vi "TPNT_file2fits.vi"(7 "mext":bool, 8 "error in (no error)":errorcluster, 9 "action":T1(ring)=enum."get all", 10 "number of Extensions":u16, 11 "filename":path=path "/home/bonati/panview_current/fpas/_decam45/config/TPNT_INFO.tpl") -> (0 "error out":errorcluster, 1 "flat keys":string[][](table), 2 "number of keywords":i32[](array[numeric]), 3 "Keywords":string[][][](array[string]), 5 "number of Extensions out":u16)   [LabVIEW 2016]
doc: "test"
panel:
  out "Extensions":i32[][](array[numeric])
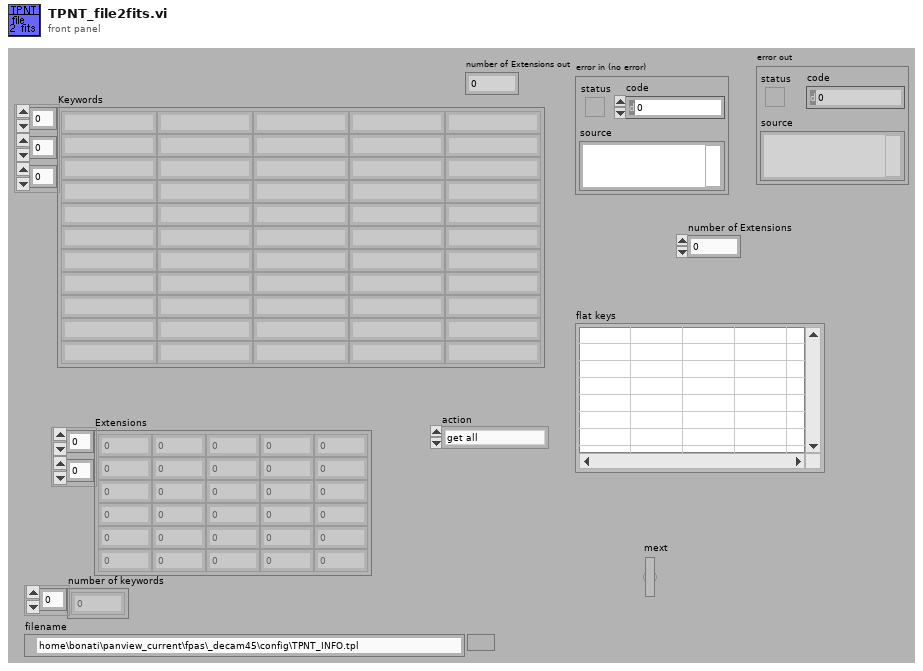
[diagram p1: front panel]
types:
  T1 = enum16{"read from file", "get all", "clear all", "set file"}
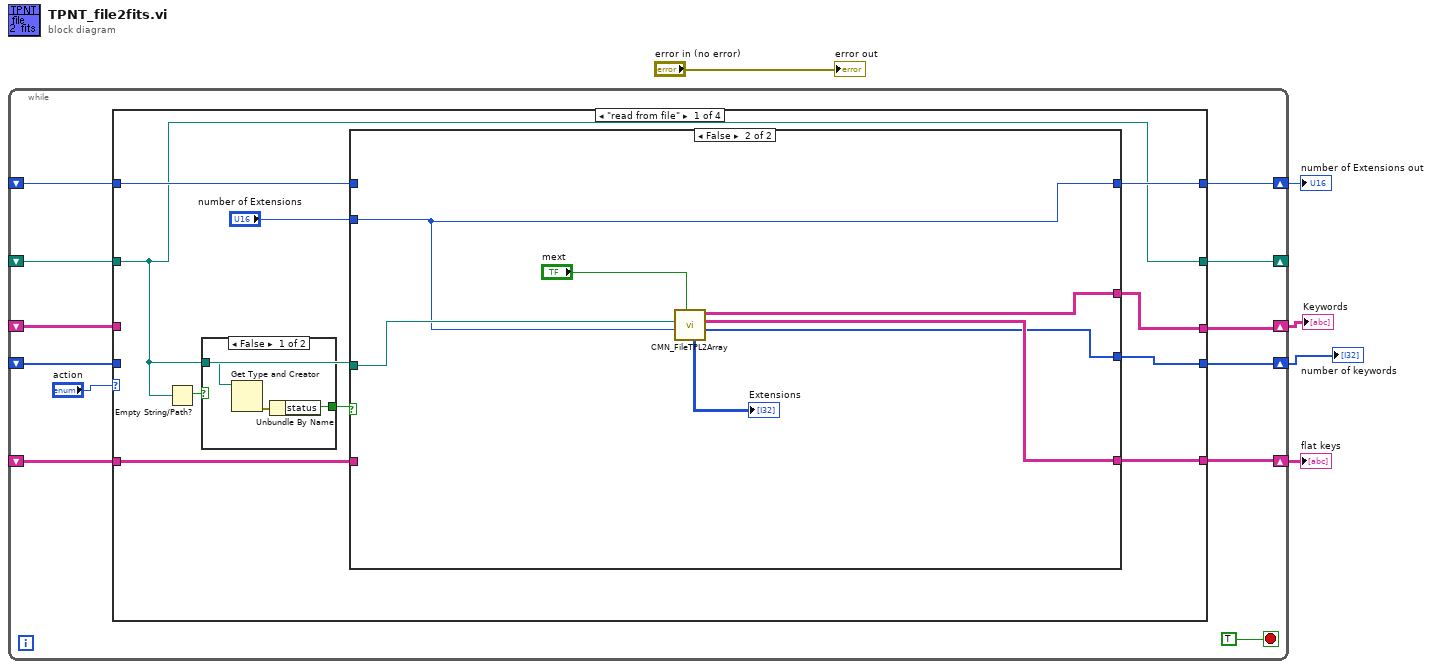
[diagram p0: block diagram]
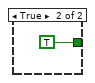
[diagram p2: hidden frame]
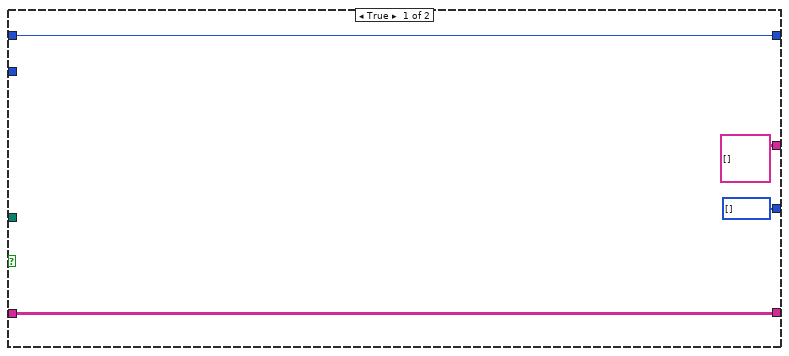
[diagram p3: hidden frame]
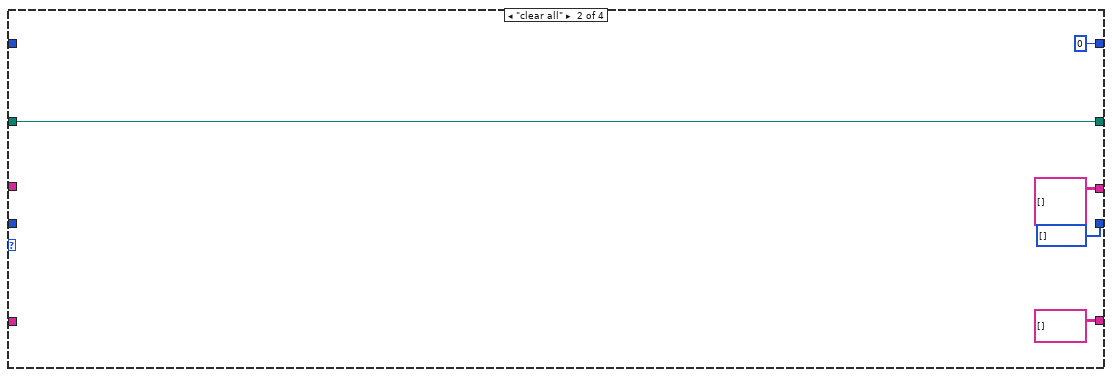
[diagram p4: hidden frame]
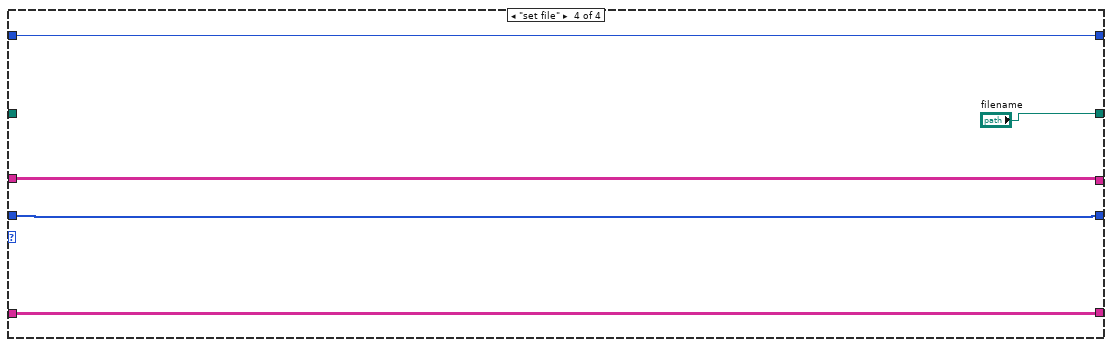
[diagram p6: hidden frame]
diagram:
  n1 = while {
    shift-right: [w16] -> w4
    shift-left: _ -> [w13]
    shift-right: [w15] -> w5
    shift-left: _ -> [w12]
    shift-right: [w11] -> w3
    shift-left: _ -> [w10]
    shift-right: [w9] -> w2
    shift-left: _ -> [w8]
    shift-right: [w7] -> _
    shift-left: _ -> [w6]
    stop <- TRUE stop-if-true
    n2 = case shown="\"read from file\"" "action" {
      tunnel: [w25 string[][][] [] w52 w57] -> w16
      tunnel: [w24 i32[] [] w51 w56] -> w15
      tunnel: w13 -> [_ _ w52 w57]
      tunnel: w12 -> [_ _ w51 w56]
      tunnel: [w23 string[][] [] w50 w55] -> w11
      tunnel: w10 -> [w22 _ w50 w55]
      tunnel: [w21 u16 0 ("number of Extensions") w49 w54] -> w9
      tunnel: w8 -> [w20 _ w49 w54]
      tunnel: [w19 w43 w48 "filename"] -> w7
      tunnel: w6 -> [w19 w43 w48 _]
      frame "read from file" {
        n3 = Empty String/Path?(string/path=w19) -> (empty?=w26:bool)
        n4 = case shown="False" w26 {
          tunnel: [w29 TRUE ("status")] -> w27
          tunnel: w19 -> [w28 _]
          frame False {
            n5 = Get Type and Creator(7:w28) -> (0:w30:errorcluster)  [unwired: 1 in, 3 out]
            n6 = Unbundle By Name(w30) -> ("status"=w29:bool)
          }
          frame True {
          }
        }
        n7 = case shown="False" w27 {
          tunnel: w19 -> [_ w42]
          tunnel: [string[][][] [] w41] -> w25
          tunnel: [i32[] [] w39] -> w24
          tunnel: [w33 w40] -> w23
          tunnel: w22 -> [w33 _]
          tunnel: [w32 w37] -> w21
          tunnel: w20 -> [w32 _]
          tunnel: "number of Extensions" -> [_ w37]
          frame True {
            (unwired) string[][] []
            (unwired) 0
          }
          frame False {
            n8 = call "CMN_FileTPL2Array.vi"("mext"="mext", "number of Extensions"=w37, "filename"=w42) -> ("number of keys"=w39:i32[], "flat keys"=w40:string[][], "Keys"=w41:string[][][], "Extensions"=→"Extensions":i32[][])  [unwired: 1 in, 4 out]
          }
        }
      }
      frame "clear all" {
      }
      frame "get all", Default {
      }
      frame "set file" {
      }
    }
  }
  "Keywords" <- w4
  "number of keywords" <- w5
  "flat keys" <- w3
  "number of Extensions out" <- w2
  "error out" <- "error in (no error)"
